vi "remove_compression_policy.vi"(7 "connection_reference":T1, 8 "error in (no error)":errorcluster, 10 "if_exists":bool, 11 "hyper_table_name":string) -> (0 "error out":errorcluster)   [LabVIEW 2015, in "lv-timescaledb.lvlib"]
uses:
  lv-timescaledb.lvlib
  <vilib>/addons/database/Connection.llb/Conn ObjectReference.ctl
  <vilib>/addons/database/Command.llb/Cmd Execute.vi
  <vilib>/addons/database/Recordset.llb/Rec Destroy - Command.vi
  <vilib>/addons/database/Command.llb/Cmd Delete.vi
  <vilib>/addons/database/NI_Database_API.lvlib
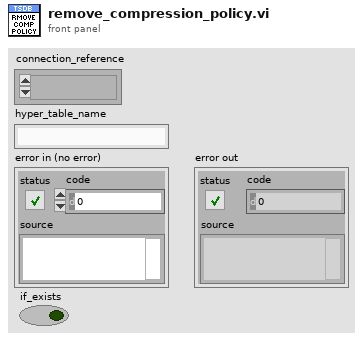
[diagram p1: front panel]
types:
  T1 = typedef "NI_Database_API.lvlib/Conn ObjectReference.ctl" = refnum<k1>
  T2 = cluster{"hyper_table_name":string, "if_exists":bool}
  T3 = typedef "NI_Database_API.lvlib/DB Tools Parameter Info.ctl" = cluster{"parameter name":string, "type":T4, "direction":T5, "value":variant}
  T4 = typedef "NI_Database_API.lvlib/DB Tools DataTypes.ctl" = enum16{"String", "Long (I32)", "Single (SGL)", "Double (DBL)", "Date/Time", "Binary"}
  T5 = typedef "NI_Database_API.lvlib/DB Tools Parameter Dir.ctl" = enum32{"Input", "Output", "Input/Output", "Return Value"}
  T6 = typedef "NI_Database_API.lvlib/Cmd ObjectReference.ctl" = refnum<k1>
  T7 = typedef "NI_Database_API.lvlib/Cmd-Rec Object Reference.ctl" = refnum<k1>
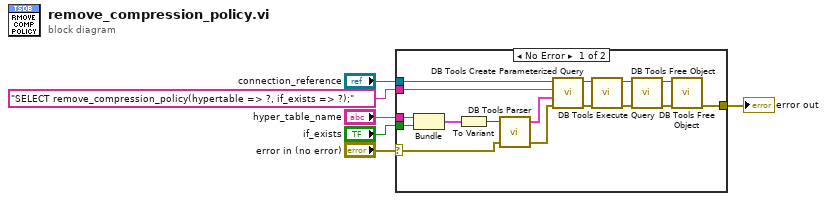
[diagram p0: block diagram]
diagram:
  n1 = case shown="No Error" "error in (no error)" {
    selector: "error in (no error)" -> [w11 w23]
    tunnel: "hyper_table_name" -> [w15 _]
    tunnel: "connection_reference" -> [w9 _]
    tunnel: [w7 w23] -> w3
    tunnel: "SELECT remove_compression_policy(hypertable => ?, if_exists => ?);" -> [w8 _]
    tunnel: "if_exists" -> [w14 _]
    frame No Error {
      n2 = Bundle("hyper_table_name"=w15, "if_exists"=w14) -> (w13:T2)  [unwired: 1 in]
      n3 = To Variant(anything=w13) -> (Variant=w12:variant)
      n4 = call <vilib>:"DB Tools Parser.vi"("error in (no error)"=w11, "variant"=w12) -> ("error out"=w10:errorcluster, "parameters"=w22:T3[])  [unwired: 2 in]
      n5 = call <vilib>:"DB Tools Create Parameterized Query.vi"("error in (no error)"=w10, "parameters"=w22, "SQL query"=w8, "connection reference"=w9) -> ("error out"=w17:errorcluster, "command reference"=w19:T6)  [unwired: 3 in, 1 out]
      n6 = call-poly <vilib>:"DB Tools Execute Query.vi"("error in (no error)"=w17, "command reference"=w19) -> ("error out"=w16:errorcluster, "command-recordset reference"=w20:T7)  [unwired: 6 in]
      n7 = call-poly <vilib>:"DB Tools Free Object.vi"("error in (no error)"=w16, "command-recordset reference"=w20) -> ("error out"=w18:errorcluster, "command reference"=w21:T6)  [unwired: 8 in]
      n8 = call-poly <vilib>:"DB Tools Free Object.vi"("error in (no error)"=w18, "command reference"=w21) -> ("error out"=w7:errorcluster)  [unwired: 8 in, 1 out]
    }
    frame Error {
    }
  }
  "error out" <- w3
